vi "Power Peak Data Acquisition.vi"() -> (0 "df":dbl, 1 "Calibration Data":dbl[](array[numeric]))   [LabVIEW 2013]
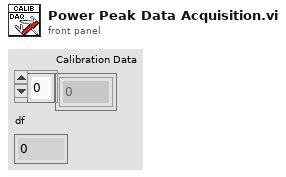
[diagram p1: front panel]
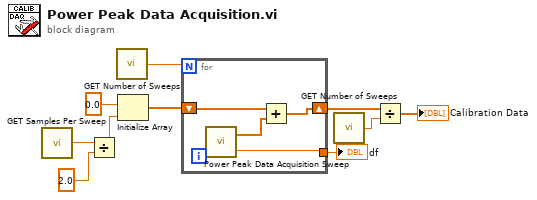
[diagram p0: block diagram]
diagram:
  n1 = call "GET Samples Per Sweep.vi"() -> ("Samples Per Sweep"=w6:dbl)
  n2 = Divide(x=w6, y=2.0) -> (x/y=w7:dbl)
  n3 = call "GET Number of Sweeps.vi"() -> ("Number of Sweeps"=w10:dbl)
  n4 = Initialize Array(0.0, w7) -> (w5:dbl[])
  n5 = for {
    N: w10 -> [_]
    shift-right: [w12] -> w3
    shift-left: w5 -> [w14]
    tunnel: [w11] -> w1
    n6 = call "Power Peak Data Acquisition Sweep.vi"() -> ("df"=w11:dbl, "Power Spectrum (V^2 rms)"=w13:dbl[])  [unwired: 2 in]
    n7 = Add(x=w14, y=w13) -> (x+y=w12:dbl[])
  }
  "df" <- w1
  n8 = call "GET Number of Sweeps.vi"() -> ("Number of Sweeps"=w4:dbl)
  n9 = Divide(x=w3, y=w4) -> (x/y=→"Calibration Data":dbl[])
